vi "Calculate Particle Scores2.vi"(10 "Sorted Data":dbl[][](array[numeric])) -> (3 "Scores":T1[](array[typedef]))   [LabVIEW 2025]
doc: "Calculate scores based on the particle measurements. Calculated scores are for aspect ratio, area to convex hull area, and moment of inertia. These scores range between 0 and 100 and can be used to categorize particles as targets and non-targets."
uses:
  Target Fields.ctl
  <vilib>/Analysis/baseanly.llb/Mean (DBL).vi
  <vilib>/Analysis/NI_AALBase.lvlib
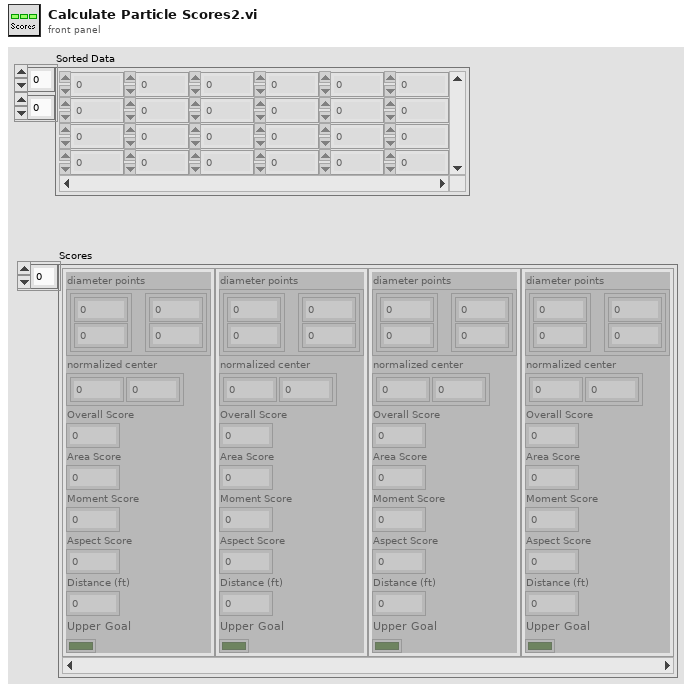
[diagram p1: front panel]
types:
  T1 = typedef "Target Fields.ctl" = cluster{"diameter points":cluster{"first point":cluster{"x":dbl, "y":dbl}, "projected point":cluster{"x":dbl, "y":dbl}}, "normalized center":cluster{"x":dbl, "y":dbl}, "Overall Score":dbl, "Area Score":dbl, "Moment Score":dbl, "Aspect Score":dbl, "Distance (ft)":dbl, "Upper Goal":bool}
  T2 = cluster{cluster{"Numeric":dbl, "Numeric":dbl}, cluster{"Numeric":dbl, "Numeric":dbl}}
  T3 = cluster{"first point":cluster{"x":dbl, "y":dbl}, "projected point":cluster{"x":dbl, "y":dbl}}
  T4 = cluster{cluster{"first point":cluster{"x":dbl, "y":dbl}, "projected point":cluster{"x":dbl, "y":dbl}}, "first point":cluster{"x":dbl, "y":dbl}, "mean":dbl, "Score":dbl, "Score":dbl, "Score":dbl, dbl, bool}
  T5 = cluster{cluster{cluster{"Numeric":dbl, "Numeric":dbl}, cluster{"Numeric":dbl, "Numeric":dbl}}, "first point":cluster{"x":dbl, "y":dbl}, "mean":dbl, "Score":dbl, "Score":dbl, "Score":dbl, dbl, bool}
  T6 = cluster{cluster{"first point":cluster{"Numeric":dbl, "Numeric":dbl}, "projected point":cluster{"Numeric":dbl, "Numeric":dbl}}, "first point":cluster{"x":dbl, "y":dbl}, "mean":dbl, "Score":dbl, "Score":dbl, "Score":dbl, dbl, bool}
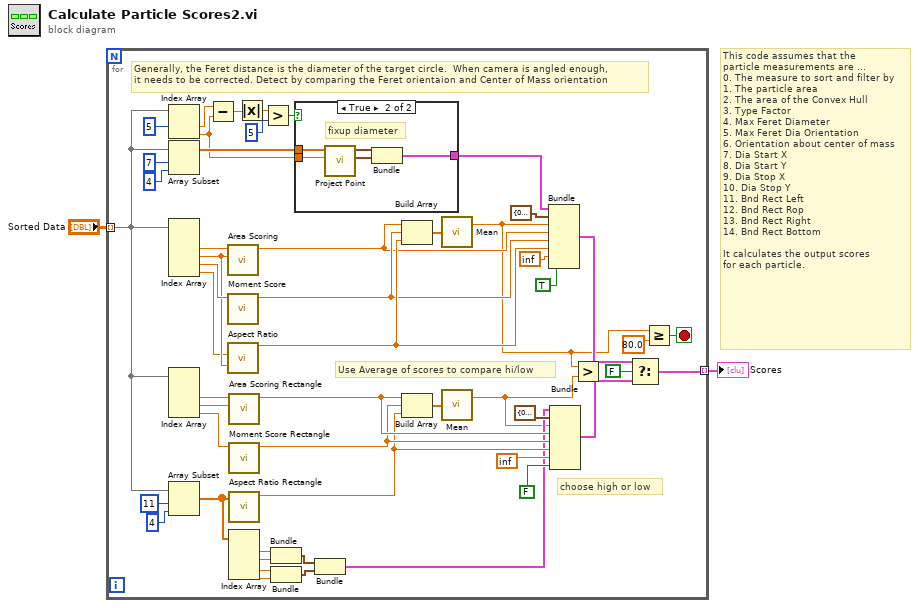
[diagram p0: block diagram]
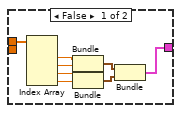
[diagram p2: hidden frame]
diagram:
  # "This code assumes that the\nparticle measurements are ...\n0. The measure to sort and filter by\n1. The particle area\n2. The area of the Convex Hull\n3. Type Factor\n4. Max Feret Diameter\n5. Max Feret Dia Orientation\n6. Orientation about center of mass\n7. Dia Start X\n8. Dia Start Y\n9. Dia Stop X\n10. Dia Stop Y\n11. Bnd Rect Left\n12. Bnd Rect Rop\n13. Bnd Rect Right\n14. Bnd Rect Bottom\n\nIt calculates the output scores\nfor each particle."
  n1 = for {
    tunnel: "Sorted Data" -> [w11] mode=indexing
    tunnel: [w25] -> w1 mode=indexing
    stop <- w7 stop-if-true
    # "Use Average of scores to compare hi/low"
    # "choose high or low"
    # "Generally, the Feret distance is the diameter of the target circle.  When camera is angled enough,\nit needs to be corrected. Detect by comparing the Feret orientaion and Center of Mass orientation"
    n2 = Index Array(array=w11, index #1=5 ("index")) -> (element #1=w46:dbl, element #2=w41:dbl)  [unwired: 1 in]
    n3 = Array Subset(array=w11, index=7, length=4) -> (w42:dbl[])
    n4 = Index Array(array=w11) -> (element #2=w53:dbl, element #3=w51:dbl, element #4=w52:dbl, element #5=w50:dbl)  [unwired: 5 in, 1 out]
    n5 = Index Array(array=w11) -> (element #2=w32:dbl, element #3=w31:dbl, element #4=w30:dbl)  [unwired: 4 in, 1 out]
    n6 = Array Subset(array=w11, index=11, length=4) -> (w10:dbl[])
    n7 = Subtract(x=w46, y=w41) -> (x-y=w49:dbl)
    n8 = call "Area Scoring.vi"("Convex Hull Area"=w51, "Area"=w53) -> ("Score"=w36:dbl)  [unwired: 9 in]
    n9 = call "Moment Score.vi"("Moment Factor"=w52) -> ("Score"=w37:dbl)  [unwired: 10 in]
    n10 = call "Aspect Ratio.vi"("Diameter"=w50, "Convex Hull Area"=w51) -> ("Score"=w38:dbl)  [unwired: 9 in]
    n11 = call "Area Scoring Rectangle.vi"("Convex Hull Area"=w31, "Area"=w32) -> ("Score"=w23:dbl)  [unwired: 9 in]
    n12 = call "Moment Score Rectangle.vi"("Moment Factor"=w30) -> ("Score"=w22:dbl)  [unwired: 10 in]
    n13 = call "Aspect Ratio Rectangle.vi"("Bounds"=w10) -> ("Score"=w21:dbl)  [unwired: 10 in]
    n14 = Index Array(array=w10) -> (element #1=w18:dbl, element #2=w17:dbl, element #3=w16:dbl, element #4=w15:dbl)  [unwired: 4 in]
    n15 = Absolute Value(x=w49) -> (abs(x)=w47:dbl)
    n16 = Greater?(x=w47, y=5 ("length")) -> (0:w40:bool)
    n17 = Bundle("Numeric"=w18, "Numeric"=w17) -> (w14:cluster{"Numeric":dbl, "Numeric":dbl})  [unwired: 1 in]
    n18 = Bundle("Numeric"=w16, "Numeric"=w15) -> (w13:cluster{"Numeric":dbl, "Numeric":dbl})  [unwired: 1 in]
    n19 = case shown="True" w40 {
      tunnel: w42 -> [w59 w66]
      tunnel: w41 -> [_ w65]
      tunnel: [w54 w62] -> w35
      frame False {
        n20 = Index Array(array=w59) -> (element #1=w57:dbl, element #2=w58:dbl, element #3=w60:dbl, element #4=w61:dbl)  [unwired: 4 in]
        n21 = Bundle("Numeric"=w57, "Numeric"=w58) -> (w56:cluster{"Numeric":dbl, "Numeric":dbl})  [unwired: 1 in]
        n22 = Bundle("Numeric"=w60, "Numeric"=w61) -> (w55:cluster{"Numeric":dbl, "Numeric":dbl})  [unwired: 1 in]
        n23 = Bundle(w56, w55) -> (w54:T2)  [unwired: 1 in]
      }
      frame True {
        # "fixup diameter"
        n24 = call "Project Point.vi"("orientation (deg)"=w65, "coordinates"=w66) -> ("projected point"=w63:cluster{"x":dbl, "y":dbl}, "first point"=w64:cluster{"x":dbl, "y":dbl})  [unwired: 8 in]
        n25 = Bundle("first point"=w64, "projected point"=w63) -> (w62:T3)  [unwired: 1 in]
      }
    }
    n26 = Bundle(w14, w13) -> (w12:T2)  [unwired: 1 in]
    n27 = Build Array(w36, w37, w38) -> (w6:dbl[])
    n28 = Build Array(w23, w22, w21) -> (w5:dbl[])
    n29 = call-poly <vilib>:"Mean.vi"("X"=w6) -> ("mean"=w9:dbl)  [unwired: 1 out]
    n30 = call-poly <vilib>:"Mean.vi"("X"=w5) -> ("mean"=w4:dbl)  [unwired: 1 out]
    n31 = Bundle(w35, "first point"=cluster{"x":dbl, "y":dbl} {"x"=0.0, "y"=0.0}, "mean"=w9, "Score"=w36, "Score"=w37, "Score"=w38, inf, TRUE) -> (w26:T4)  [unwired: 1 in]
    n32 = Bundle(w12, "first point"=cluster{"x":dbl, "y":dbl} {"x"=0.0, "y"=0.0}, "mean"=w4, "Score"=w23, "Score"=w22, "Score"=w21, inf, FALSE) -> (w27:T5)  [unwired: 1 in]
    n33 = Greater?(x=w9, y=w4) -> ()  [unwired: 1 out]
    n34 = Select(t=w26, s=FALSE, f=w27) -> (s? t:f=w25:T6)
    n35 = Greater Or Equal?(x=w9, y=80.0) -> (x >= y?=w7:bool)
  }
  "Scores" <- w1
